vi "Create Message Setter (from Template).vi"(8 "error in (no error)":errorcluster, 10 "RPC Message Name":string, 11 "RPC Messages Folder (ProjectItem) in":refnum<vi>) -> (0 "error out":errorcluster, 1 "Created?":bool, 2 "VI out":refnum<vi>, 3 "RPC Messages Folder (ProjectItem) out":refnum<vi>)   [LabVIEW 2019, in "gRPC Scripting Tools.lvlib"]
uses:
  gRPC Scripting Tools.lvlib
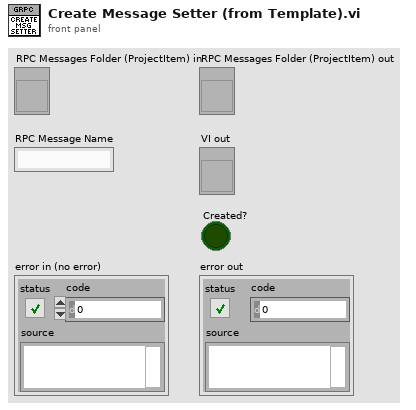
[diagram p1: front panel]
types:
  T1 = enum32{"invalid VI type", "Standard VI", "Control VI", "Global VI", "Polymorphic VI", "Configuration VI", "SubSystem", "Facade VI", "Method VI"}
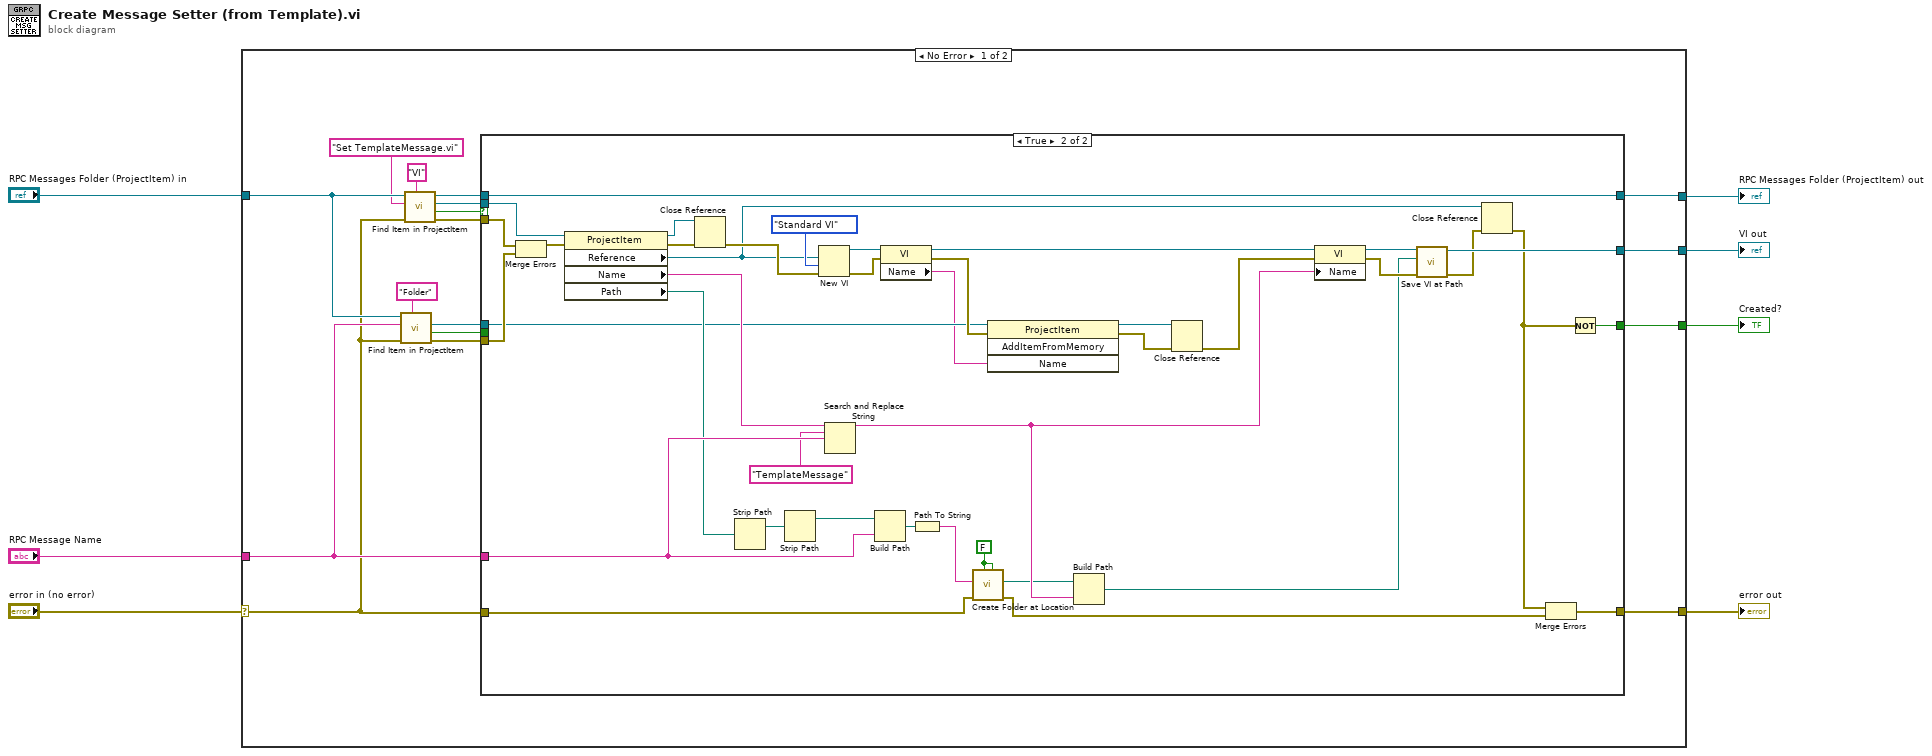
[diagram p0: block diagram]
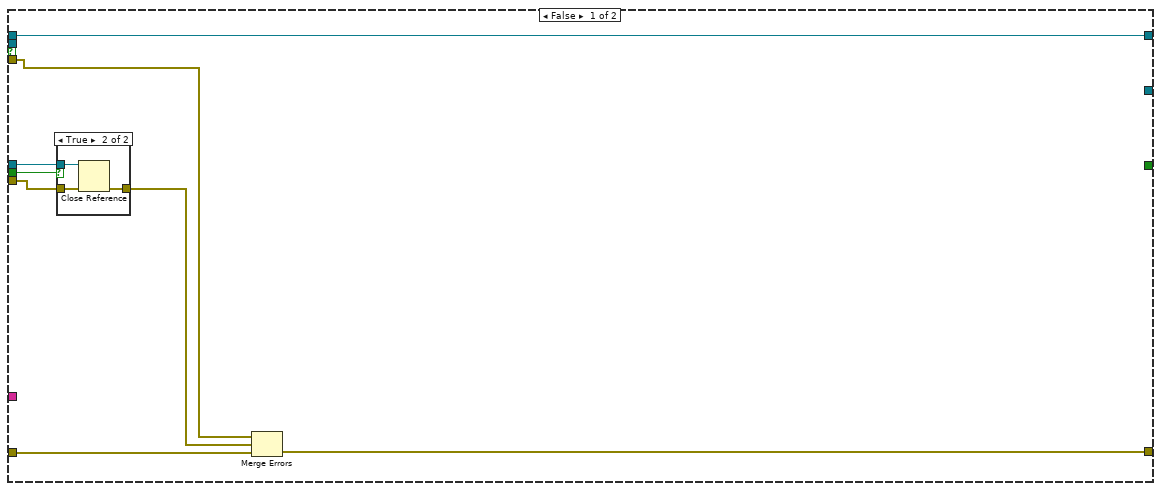
[diagram p2: hidden frame]
diagram:
  n1 = case shown="No Error" "error in (no error)" {
    selector: "error in (no error)" -> [w13 w77]
    tunnel: "RPC Message Name" -> [w24 _]
    tunnel: "RPC Messages Folder (ProjectItem) in" -> [w23 w78]
    tunnel: [w22 w77] -> w5
    tunnel: [w10 w78] -> w4
    tunnel: [w19 _] -> w3
    tunnel: [w9 _] -> w1
    frame No Error {
      n2 = call "Find Item in ProjectItem.vi"("Item Type"="Folder", "error in (no error)"=w13, "Name"=w24, "ProjectItem in"=w23) -> ("error out"=w21:errorcluster, "Found ?"=w8:bool, "Item Refnum out"=w18:refnum<vi>)  [unwired: 4 in, 1 out]
      n3 = call "Find Item in ProjectItem.vi"("Item Type"="VI", "error in (no error)"=w13, "Name"="Set TemplateMessage.vi", "ProjectItem in"=w23) -> ("error out"=w20:errorcluster, "Found ?"=w12:bool, "Item Refnum out"=w17:refnum<vi>, "ProjectItem out"=w11:refnum<vi>)  [unwired: 4 in]
      n4 = case shown="True" w12 {
        tunnel: w24 -> [_ w76]
        tunnel: [w27 w72] -> w22
        tunnel: w21 -> [w31 w70]
        tunnel: w20 -> [w26 w68]
        tunnel: [_ w66] -> w19
        tunnel: w18 -> [w30 w51]
        tunnel: w17 -> [_ w46]
        tunnel: w13 -> [w28 w45]
        tunnel: w11 -> [w32 w44]
        tunnel: [w32 w44] -> w10
        tunnel: [_ w40] -> w9
        tunnel: w8 -> [w25 _]
        frame False {
          n5 = case shown="True" w25 {
            tunnel: w31 -> [w33 w36]
            tunnel: w30 -> [_ w35]
            tunnel: [w33 w34] -> w29
            frame False {
            }
            frame True {
              n6 = Close Reference(reference=w35, error in (no error)=w36) -> (error out=w34:errorcluster)
            }
          }
          n7 = Merge Errors(w26, w29, w28) -> (w27:errorcluster)
        }
        frame True {
          w67 = FALSE ("Use Relative (F)")
          n8 = Merge Errors(w68, w70) -> (w69:errorcluster)
          n9 = property class="ProjectItem"(reference=w46, error in=w69) -> (reference out=w75:refnum<vi>, error out=w73:errorcluster, "Reference"=w37:refnum<vi>, "Name"=w58:string, "Path"=w56:path)
          n10 = Close Reference(reference=w75, error in (no error)=w73) -> (error out=w74:errorcluster)
          n11 = Strip Path(path=w56) -> (stripped path=w52:path)  [unwired: 1 out]
          n12 = Strip Path(path=w52) -> (stripped path=w53:path)  [unwired: 1 out]
          n13 = New VI(8:w74, 9:T1."Standard VI" ("vi type (standard vi)"), 10:w37) -> (0:w49:errorcluster, 3:w47:refnum<vi>)  [unwired: 1 in, 3 out]
          n14 = Search and Replace String(input string=w58, search string="TemplateMessage", replace string=w76) -> (result string=w62:string)  [unwired: 5 in, 3 out]
          n15 = Build Path(base path=w53, name or relative path=w76) -> (appended path=w54:path)
          n16 = property class="VI"(reference=w47, error in=w49) -> (reference out=w59:refnum<vi>, error out=w60:errorcluster, "Name"=w50:string)
          n17 = Path To String(path=w54) -> (string=w55:string)
          n18 = call "Create Folder at Location.vi"("Override existing (F)"=w67, "Use Relative (F)"=w67, "Error In"=w45, "Path"=w55) -> ("Error Out"=w71:errorcluster, "Full path out"=w61:path)  [unwired: 5 in, 1 out]
          n19 = invoke class="ProjectItem" method="AddItemFromMemory"(reference=w51, error in=w60, "Name"=w50) -> (reference out=w42:refnum<vi>, error out=w43:errorcluster)  [unwired: 1 in, 2 out]
          n20 = Build Path(base path=w61, name or relative path=w62) -> (appended path=w64:path)
          n21 = Close Reference(reference=w42, error in (no error)=w43) -> (error out=w41:errorcluster)
          n22 = property class="VI"(reference=w59, error in=w41, "Name"=w62) -> (reference out=w63:refnum<vi>, error out=w65:errorcluster)
          n23 = call "Save VI at Path.vi"("error in (no error)"=w65, "Path"=w64, "VI in"=w63) -> ("error out"=w39:errorcluster, "VI out"=w66:refnum<vi>)  [unwired: 6 in, 1 out]
          n24 = Close Reference(reference=w37, error in (no error)=w39) -> (error out=w38:errorcluster)
          n25 = Merge Errors(w38, w71) -> (w72:errorcluster)
          n26 = Not(x=w38) -> (.not. x?=w40:bool)
        }
      }
    }
    frame Error {
    }
  }
  "error out" <- w5
  "RPC Messages Folder (ProjectItem) out" <- w4
  "VI out" <- w3
  "Created?" <- w1
